vi "TEST ASIC DIGITAL OFFSET FIND INIT END.vi"(10 "LVDS":bool[](array[boolean]), 11 "SCALER":u16[](array[numeric])) -> (2 "Max":i32, 3 "Min":i32)   [LabVIEW 2019]
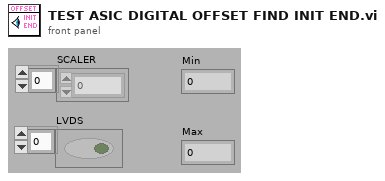
[diagram p1: front panel]
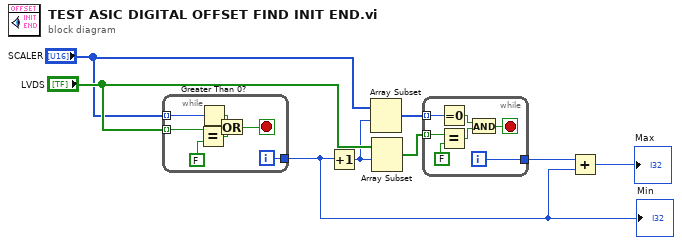
[diagram p0: block diagram]
diagram:
  n1 = while {
    tunnel: "LVDS" -> [w12] mode=indexing
    tunnel: "SCALER" -> [w11] mode=indexing
    tunnel: [w10] -> w5
    i -> [w10]
    stop <- w9 stop-if-true
    n2 = Equal?(x=w12, y=FALSE) -> (x = y?=w15:bool)
    n3 = Greater Than 0?(x=w11) -> (x > 0?=w14:bool)
    n4 = Or(x=w15, y=w14) -> (x .or. y?=w9:bool)
  }
  "Min" <- w5
  n5 = Increment(x=w5) -> (x+1=w1:i32)
  n6 = Array Subset(array="SCALER", index=w1) -> (w3:u16[])  [unwired: 1 in]
  n7 = Array Subset(array="LVDS", index=w1) -> (w4:bool[])  [unwired: 1 in]
  n8 = while {
    tunnel: w4 -> [w21] mode=indexing
    tunnel: w3 -> [w20] mode=indexing
    tunnel: [w16] -> w2
    i -> [w16]
    stop <- w17 stop-if-true
    n9 = Equal To 0?(x=w20) -> (x = 0?=w18:bool)
    n10 = Equal?(x=w21, y=FALSE) -> (x = y?=w19:bool)
    n11 = And(x=w19, y=w18) -> (x .and. y?=w17:bool)
  }
  n12 = Add(x=w2, y=w5) -> (x+y=→"Max":i32)
